vi "TestExec.Set Option Controls.vi"(8 "Disable SN Route Ck":bool, 9 "TE Opts":T2[](array[typedef]) caption="Option                                          Level", 11 "TE Opts In":T1 caption="TE Options") -> (3 "TE Opts Out":T1 caption="TE Options Out")   [LabVIEW 2018]
uses:
  Controls and Type Defs/TestExec.Options Ctrls.ctl
  Mode Manager/ModeMgr.Mode Settings.ctl
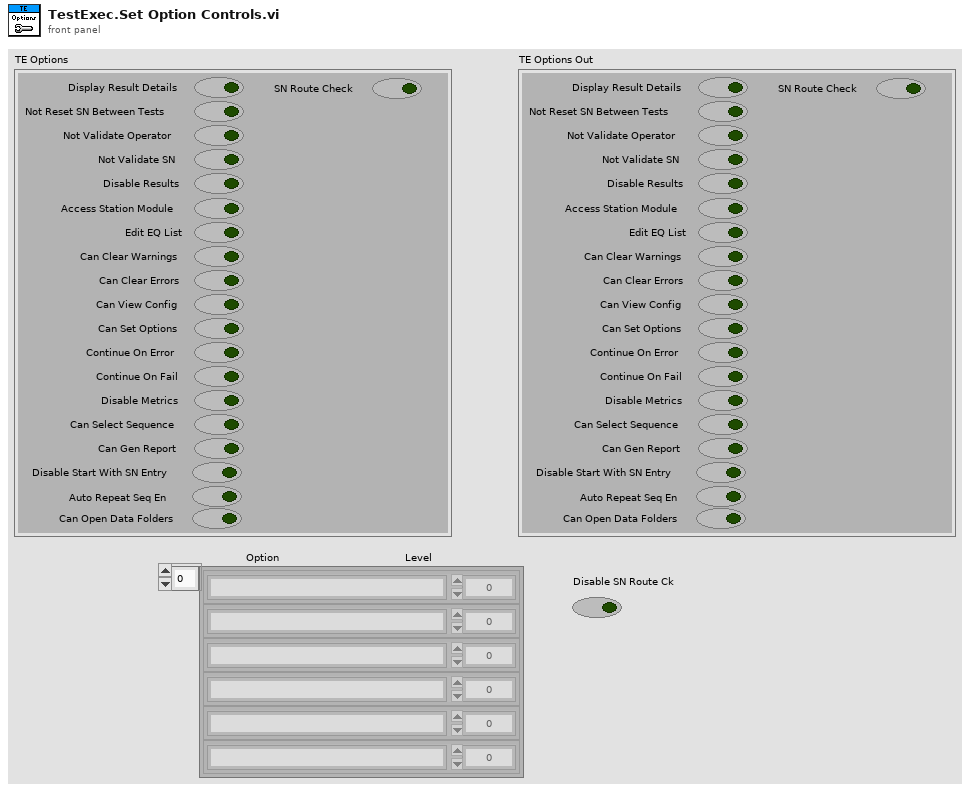
[diagram p1: front panel]
types:
  T1 = typedef "TestExec.Options Ctrls.ctl" = cluster{"DispDetails":bool, "NotResetSN":bool, "NotValOper":bool, "NotValSN":bool, "DisResults":bool, "StaModule":bool, "EditEQ":bool, "ClrWarn":bool, "ClrErr":bool, "ViewCfg":bool, "SetOpts":bool, "ContOnErr":bool, "ContOnFail":bool, "DisMetrics":bool, "SelSeq":bool, "GenRpt":bool, "DisStartWithSN":bool, "Auto Repeat Seq En":bool, "DataDirEn":bool, "SNRouteCk":bool}
  T2 = typedef "ModeMgr.Mode Settings.ctl" = cluster{"Option":string, "Level":i32}
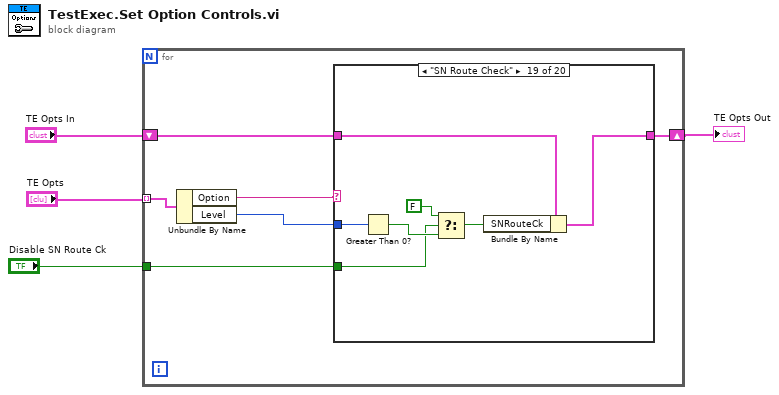
[diagram p0: block diagram]
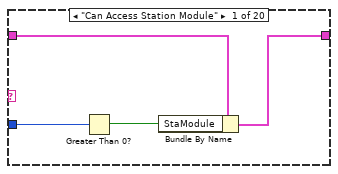
[diagram p2: hidden frame]
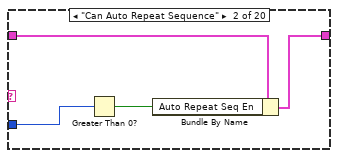
[diagram p3: hidden frame]
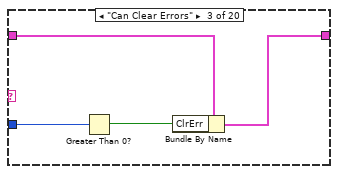
[diagram p4: hidden frame]
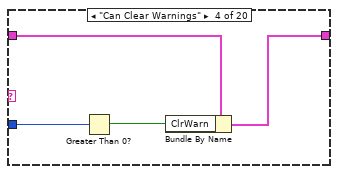
[diagram p5: hidden frame]
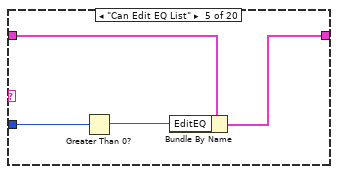
[diagram p6: hidden frame]
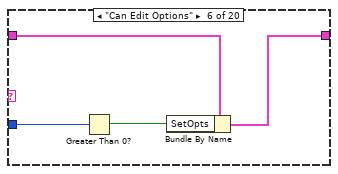
[diagram p7: hidden frame]
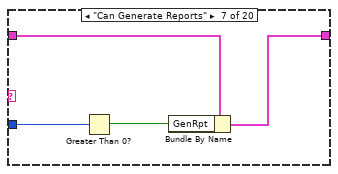
[diagram p8: hidden frame]
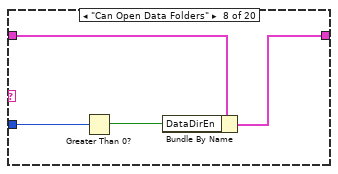
[diagram p9: hidden frame]
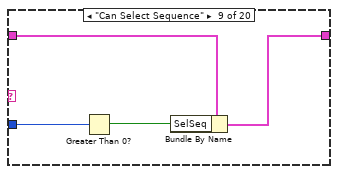
[diagram p10: hidden frame]
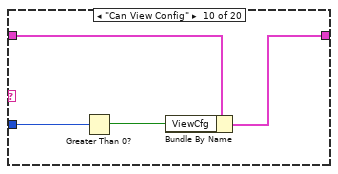
[diagram p11: hidden frame]
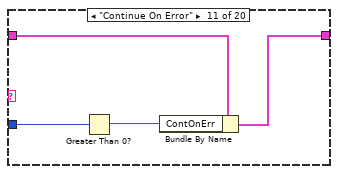
[diagram p12: hidden frame]
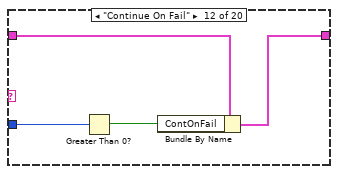
[diagram p13: hidden frame]
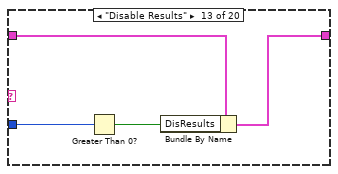
[diagram p14: hidden frame]
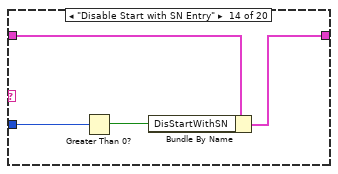
[diagram p15: hidden frame]
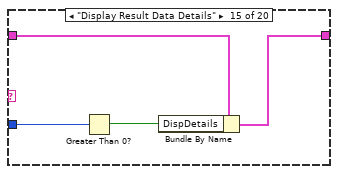
[diagram p16: hidden frame]
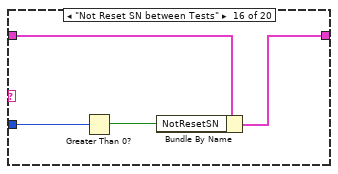
[diagram p17: hidden frame]
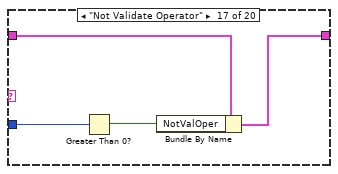
[diagram p18: hidden frame]
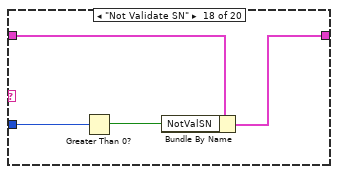
[diagram p19: hidden frame]
diagram:
  n1 = for {
    tunnel: "TE Opts" -> [w10] mode=indexing
    shift-right: [w6] -> w3
    shift-left: "TE Opts In" -> [w8]
    tunnel: "Disable SN Route Ck" -> [w5]
    n2 = Unbundle By Name(w10) -> ("Option"=w9:string, "Level"=w7:i32)
    n3 = case shown="\"SN Route Check\"" w9 {
      tunnel: w8 -> [w14 w18 w22 w26 w30 w34 w38 w42 w46 w50 w54 w58 w62 w66 w70 w74 w78 w82 w89 w90]
      tunnel: w7 -> [w13 w16 w21 w25 w29 w33 w37 w41 w45 w49 w53 w57 w59 w65 w69 w73 w77 w81 w88 _]
      tunnel: [w11 w17 w19 w23 w27 w31 w35 w39 w43 w47 w51 w55 w61 w63 w67 w71 w75 w79 w87 w90] -> w6
      tunnel: w5 -> [_ _ _ _ _ _ _ _ _ _ _ _ _ _ _ _ _ _ w85 _]
      frame "Can Access Station Module" {
        n4 = Greater Than 0?(x=w13) -> (x > 0?=w12:bool)
        n5 = Bundle By Name(cluster=w14, "StaModule"=w12) -> (w11:T1)
      }
      frame "Can Auto Repeat Sequence" {
        n6 = Greater Than 0?(x=w16) -> (x > 0?=w15:bool)
        n7 = Bundle By Name(cluster=w18, "Auto Repeat Seq En"=w15) -> (w17:T1)
      }
      frame "Can Clear Errors" {
        n8 = Greater Than 0?(x=w21) -> (x > 0?=w20:bool)
        n9 = Bundle By Name(cluster=w22, "ClrErr"=w20) -> (w19:T1)
      }
      frame "Can Clear Warnings" {
        n10 = Greater Than 0?(x=w25) -> (x > 0?=w24:bool)
        n11 = Bundle By Name(cluster=w26, "ClrWarn"=w24) -> (w23:T1)
      }
      frame "Can Edit EQ List" {
        n12 = Greater Than 0?(x=w29) -> (x > 0?=w28:bool)
        n13 = Bundle By Name(cluster=w30, "EditEQ"=w28) -> (w27:T1)
      }
      frame "Can Edit Options" {
        n14 = Greater Than 0?(x=w33) -> (x > 0?=w32:bool)
        n15 = Bundle By Name(cluster=w34, "SetOpts"=w32) -> (w31:T1)
      }
      frame "Can Generate Reports" {
        n16 = Greater Than 0?(x=w37) -> (x > 0?=w36:bool)
        n17 = Bundle By Name(cluster=w38, "GenRpt"=w36) -> (w35:T1)
      }
      frame "Can Open Data Folders" {
        n18 = Greater Than 0?(x=w41) -> (x > 0?=w40:bool)
        n19 = Bundle By Name(cluster=w42, "DataDirEn"=w40) -> (w39:T1)
      }
      frame "Can Select Sequence" {
        n20 = Greater Than 0?(x=w45) -> (x > 0?=w44:bool)
        n21 = Bundle By Name(cluster=w46, "SelSeq"=w44) -> (w43:T1)
      }
      frame "Can View Config" {
        n22 = Greater Than 0?(x=w49) -> (x > 0?=w48:bool)
        n23 = Bundle By Name(cluster=w50, "ViewCfg"=w48) -> (w47:T1)
      }
      frame "Continue On Error" {
        n24 = Greater Than 0?(x=w53) -> (x > 0?=w52:bool)
        n25 = Bundle By Name(cluster=w54, "ContOnErr"=w52) -> (w51:T1)
      }
      frame "Continue On Fail" {
        n26 = Greater Than 0?(x=w57) -> (x > 0?=w56:bool)
        n27 = Bundle By Name(cluster=w58, "ContOnFail"=w56) -> (w55:T1)
      }
      frame "Disable Results" {
        n28 = Greater Than 0?(x=w59) -> (x > 0?=w60:bool)
        n29 = Bundle By Name(cluster=w62, "DisResults"=w60) -> (w61:T1)
      }
      frame "Disable Start with SN Entry" {
        n30 = Greater Than 0?(x=w65) -> (x > 0?=w64:bool)
        n31 = Bundle By Name(cluster=w66, "DisStartWithSN"=w64) -> (w63:T1)
      }
      frame "Display Result Data Details" {
        n32 = Greater Than 0?(x=w69) -> (x > 0?=w68:bool)
        n33 = Bundle By Name(cluster=w70, "DispDetails"=w68) -> (w67:T1)
      }
      frame "Not Reset SN between Tests" {
        n34 = Greater Than 0?(x=w73) -> (x > 0?=w72:bool)
        n35 = Bundle By Name(cluster=w74, "NotResetSN"=w72) -> (w71:T1)
      }
      frame "Not Validate Operator" {
        n36 = Greater Than 0?(x=w77) -> (x > 0?=w76:bool)
        n37 = Bundle By Name(cluster=w78, "NotValOper"=w76) -> (w75:T1)
      }
      frame "Not Validate SN" {
        n38 = Greater Than 0?(x=w81) -> (x > 0?=w80:bool)
        n39 = Bundle By Name(cluster=w82, "NotValSN"=w80) -> (w79:T1)
      }
      frame "SN Route Check" {
        n40 = Greater Than 0?(x=w88) -> (x > 0?=w86:bool)
        n41 = Select(t=FALSE, s=w85, f=w86) -> (s? t:f=w83:bool)
        n42 = Bundle By Name(cluster=w89, "SNRouteCk"=w83) -> (w87:T1)
      }
      frame Default {
        # "Do nothing.\nUnrecognized Option."
      }
    }
  }
  "TE Opts Out" <- w3
